vi "Evaluate Part 1.vi"() -> ()   [LabVIEW 2020]
uses:
  Bag/Cubes.ctl
  Game/Game.lvclass
  Bag/Bag.lvclass
panel:
  in  "Input":string="Game 1: 3 blue, 4 red; 1 red, 2 green, 6 blue; 2 green\nGame 2: 1 blue, 2 green; 3 green, 4 blue, 1 red; 1 green, 1 blue\nGame 3: 8 green, 6 blue, 20 red; 5 blue, 4 red, 13 green; 5 green, 1 red\nGame 4: 1 green, 3 red, 6 blue; 3 green, 6 red; 3 green, 15 blue, 14 red\nGame 5: 6 red, 1 blue, 3 green; 2 blue, 1 red, 2 green"
  out "sum":i32=8
  out "Possible Games":i32[](array[numeric])=[1, 2, 5]
  in  "Loaded Cubes":T1={"Red"=12, "Green"=13, "Blue"=14}
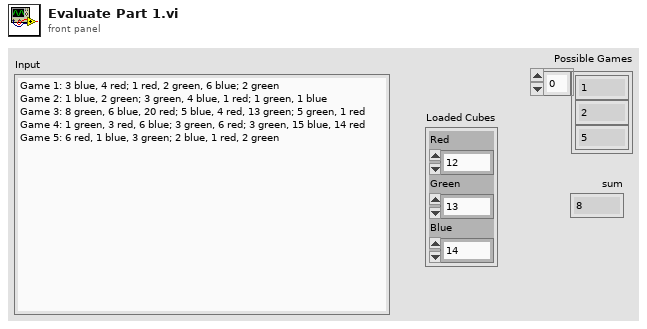
[diagram p1: front panel]
types:
  T1 = typedef "Bag.lvclass/Cubes.ctl" = cluster{"Red":i32, "Green":i32, "Blue":i32}
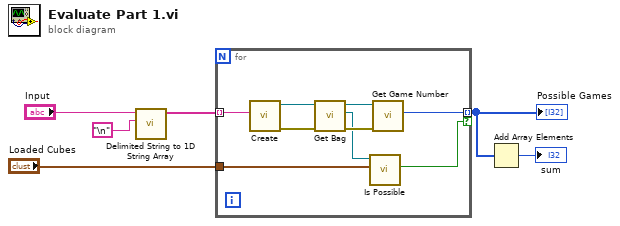
[diagram p0: block diagram]
diagram:
  n1 = call <vilib>:"Delimited String to 1D String Array.vi"("delimiter"="\n", "delimited string"="Input") -> ("string array"=w1:string[])  [unwired: 9 in]
  n2 = for {
    tunnel: "Loaded Cubes" -> [w10]
    tunnel: [w9] -> w5 mode=indexing if=w8
    tunnel: w1 -> [w7] mode=indexing
    n3 = call "Create.vi"("Input"=w7) -> ("error out"=w14:errorcluster, "Game"=w15:refnum<class "Game.lvclass">)  [unwired: 9 in]
    n4 = call "Get Bag.vi"("error in (no error)"=w14, "Game in"=w15) -> ("error out"=w12:errorcluster, "Bag"=w11:refnum<class "Bag.lvclass">, "Game out"=w13:refnum<class "Game.lvclass">)  [unwired: 7 in]
    n5 = call "Is Possible.vi"("Cubes"=w10, "Bag in"=w11) -> ("Compatible?"=w8:bool)  [unwired: 7 in, 2 out]
    n6 = call "Get Game Number.vi"("error in (no error)"=w12, "Game in"=w13) -> ("Number"=w9:i32)  [unwired: 7 in, 2 out]
  }
  "Possible Games" <- w5
  n7 = Add Array Elements(numeric array=w5) -> (sum=→"sum":i32)
